vi "Test_ConstructBinding_InvalidRefnum_Error.vi"(8 "error in (no error)":errorcluster, 11 "TestCase in":refnum<class "TestTerminalCaptionBinding.lvclass">) -> (0 "error out":errorcluster, 3 "TestCase out":refnum<class "TestTerminalCaptionBinding.lvclass">)   [LabVIEW 2017, in "TestTerminalCaptionBinding.lvclass"]
uses:
  TestTerminalCaptionBinding.lvclass
  Source/Concrete/TerminalCaptionBinding/TerminalCaptionBinding.lvclass
panel:
  out "Return Error":errorcluster
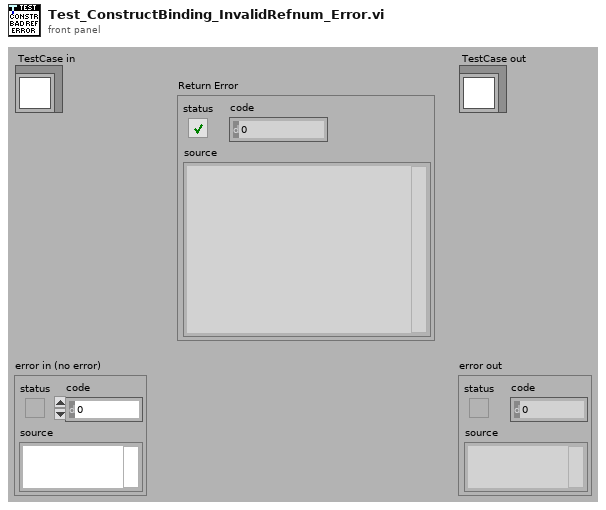
[diagram p1: front panel]
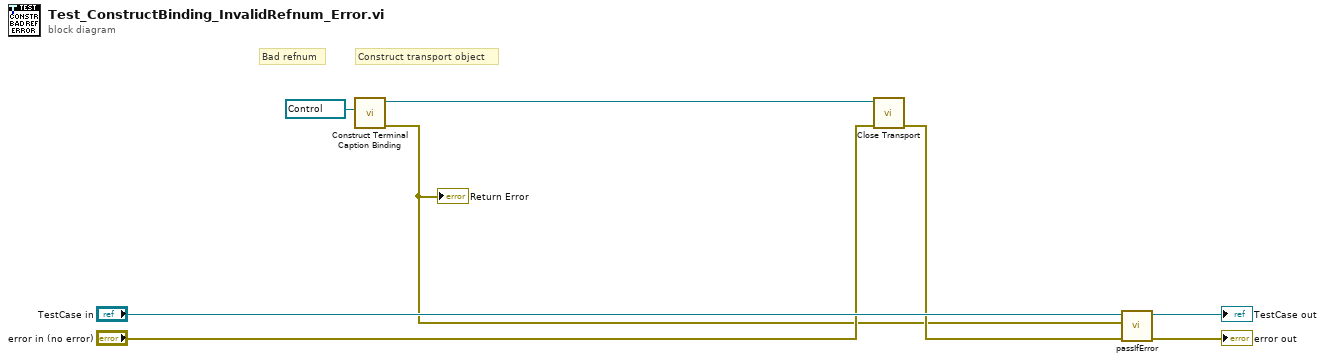
[diagram p0: block diagram]
diagram:
  # "Bad refnum"
  # "Construct transport object"
  n1 = call "Construct Terminal Caption Binding.vi"("Ctl Refnum"=refnum<vi> refnum) -> ("error out"=w2:errorcluster, "TerminalCaptionBinding"=w5:refnum<class "TerminalCaptionBinding.lvclass">)  [unwired: 9 in]
  "Return Error" <- w2
  n2 = call-dynamic "Close Transport.vi"("error in (no error)"="error in (no error)", "ITransport in"=w5) -> ("error out"=w3:errorcluster)  [unwired: 9 in]
  n3 = call-dynamic "passIfError.vi"("error in (no error)"=w3, "error"=w2, "TestCase in"="TestCase in") -> ("error out"=→"error out":errorcluster, "TestCase out"=→"TestCase out":refnum<class "TestTerminalCaptionBinding.lvclass">)  [unwired: 7 in]
